vi "LeerBD.vi"(8 "error in (no error)":errorcluster) -> (0 "error out":errorcluster, 2 "BD":T1={"niv_presion_son_ref"=97.0, "Incertidumbre"="", "Tol +"="", "Tol -"="", "max_niv_ref"=97.0, "min_niv_ref"=97.0}, 3 "Prueba06 out":refnum<class "Prueba06.lvclass">)   [LabVIEW 2019, in "Prueba06.lvclass"]
uses:
  Prueba06.lvclass
  BD.ctl
  Base de Datos/SQLiteConnector/SQLiteConnection.lvclass
  Base de Datos/Base de Datos.lvclass
panel:
  in  "Tipo Equipo":enum16{"Sonometro", "Calibrador", "Dosimetro"}(ring)
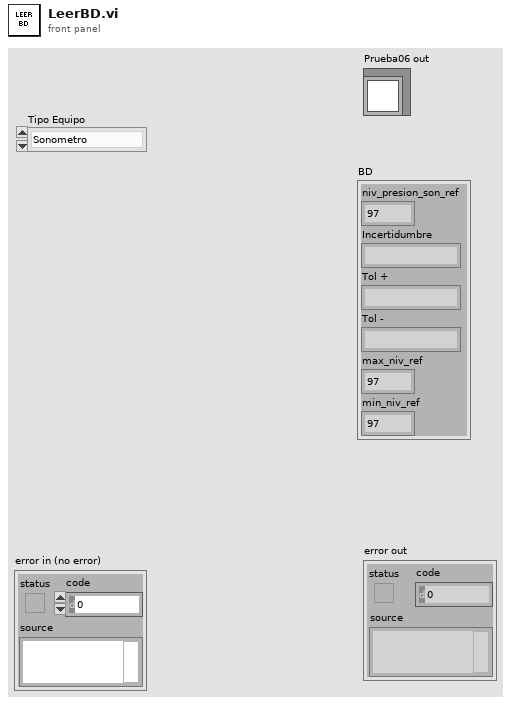
[diagram p1: front panel]
types:
  T1 = typedef "Prueba06.lvclass/BD.ctl" = cluster{"niv_presion_son_ref":dbl, "Incertidumbre":string, "Tol +":string, "Tol -":string, "max_niv_ref":dbl, "min_niv_ref":dbl}
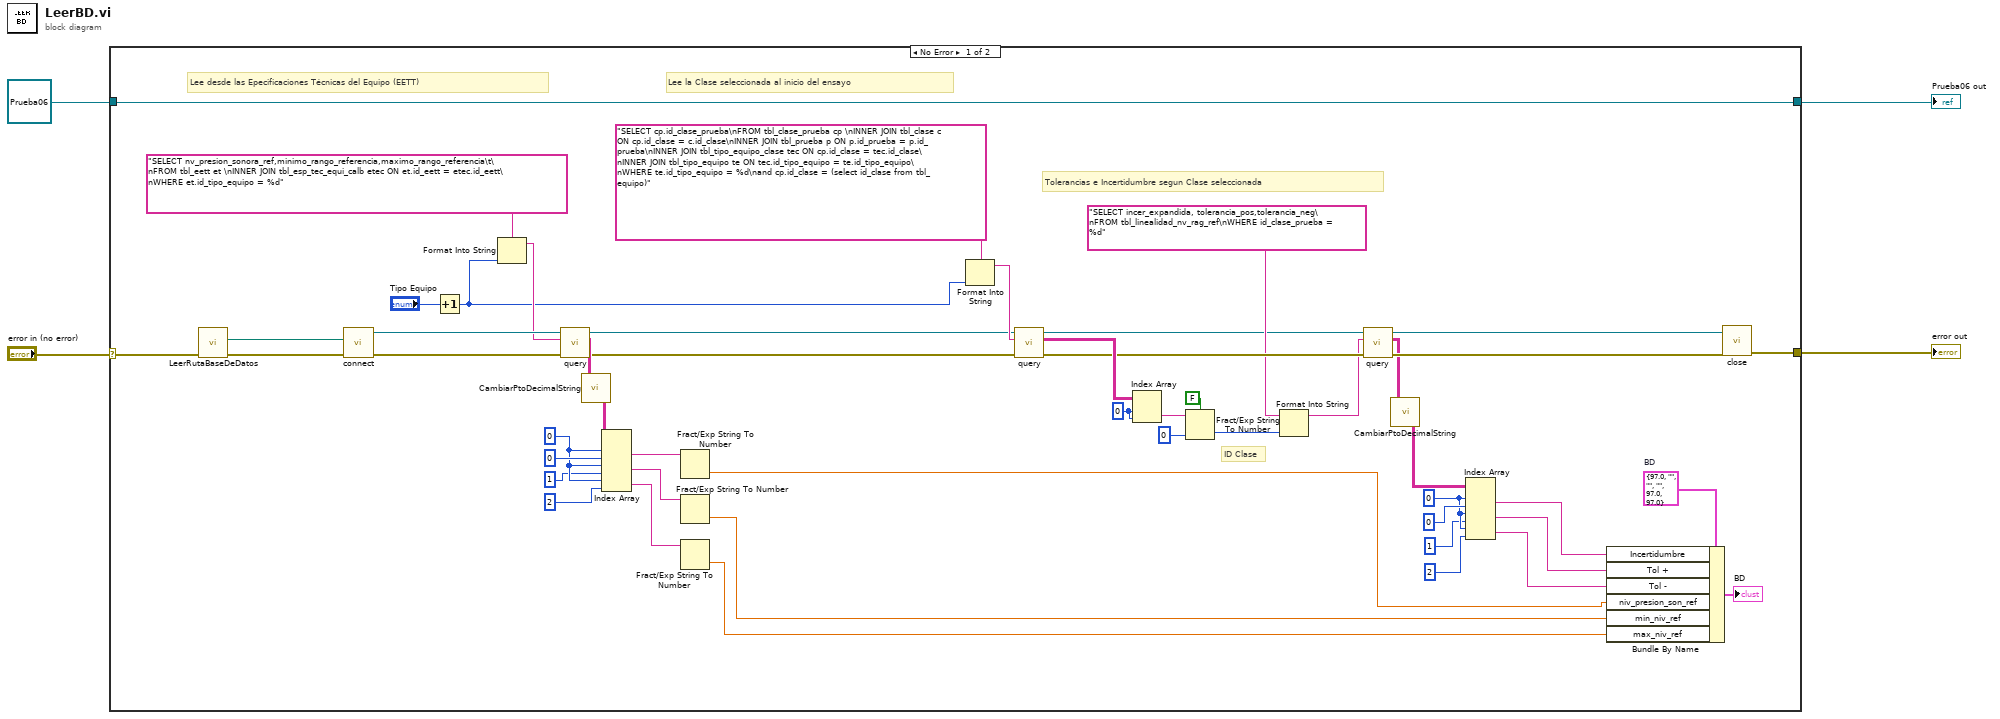
[diagram p0: block diagram]
diagram:
  n1 = case shown="No Error" "error in (no error)" {
    selector: "error in (no error)" -> [w46 w56]
    tunnel: [w32 w56] -> w3
    tunnel: [w54 w55] -> w1
    tunnel: refnum<class "Prueba06.lvclass"> refnum ("Prueba02 in") -> [w54 w55]
    frame No Error {
      w13 = 0 ("index (row)")
      w22 = T1 {"niv_presion_son_ref"=97.0, "Incertidumbre"="", "Tol +"="", "Tol -"="", "max_niv_ref"=97.0, "min_niv_ref"=97.0}  # BD
      w38 = 0 ("index (row)")
      w21 = 0 ("index (row)")
      # "Tolerancias e Incertidumbre segun Clase seleccionada"
      # "ID Clase"
      # "Lee la Clase seleccionada al inicio del ensayo"
      # "Lee desde las Epecificaciones Técnicas del Equipo (EETT)"
      n2 = call "LeerRutaBaseDeDatos.vi"("error in (no error)"=w46) -> ("error out"=w49:errorcluster, "Database Path"=w48:path)  [unwired: 9 in]
      n3 = call "connect.vi"("error in (no error)"=w49, "Database Path"=w48) -> ("error out"=w51:errorcluster, "object out"=w52:refnum<class "SQLiteConnection.lvclass">)  [unwired: 8 in]
      n4 = Increment(x="Tipo Equipo") -> (x+1=w27:enum16{"Sonometro", "Calibrador", "Dosimetro"})
      n5 = Format Into String(format string="SELECT nv_presion_sonora_ref,minimo_rango_referencia,maximo_rango_referencia\t\nFROM tbl_eett et \nINNER JOIN tbl_esp_tec_equi_calb etec ON et.id_eett = etec.id_eett\nWHERE et.id_tipo_equipo = %d", w27) -> (resulting string=w50:string)  [unwired: 2 in, 1 out]
      n6 = call "query.vi"("error in (no error)"=w51, "SQL Statement"=w50, "object in"=w52) -> ("error out"=w39:errorcluster, "result"=w43:string[][], "object out"=w40:refnum<class "SQLiteConnection.lvclass">)  [unwired: 5 in, 1 out]
      n7 = call "CambiarPtoDecimalString.vi"("result"=w43) -> ("result out"=w6:string[][])
      n8 = Index Array(array=w6, index (row) #1=w21, index (col) #1=0 ("disabled index (col)"), index (row) #2=w21, index (col) #2=1 ("disabled index (col)"), index (row) #3=w21, index (col) #3=2 ("disabled index (col)")) -> (element #1=w44:string, element #2=w18:string, element #3=w17:string)
      n9 = Fract/Exp String To Number(string=w44) -> (number=w23:dbl)  [unwired: 3 in, 1 out]
      n10 = Fract/Exp String To Number(string=w18) -> (number=w16:dbl)  [unwired: 3 in, 1 out]
      n11 = Fract/Exp String To Number(string=w17) -> (number=w15:dbl)  [unwired: 3 in, 1 out]
      n12 = Format Into String(format string="SELECT cp.id_clase_prueba\nFROM tbl_clase_prueba cp \nINNER JOIN tbl_clase c ON cp.id_clase = c.id_clase\nINNER JOIN tbl_prueba p ON p.id_prueba = p.id_prueba\nINNER JOIN tbl_tipo_equipo_clase tec ON cp.id_clase = tec.id_clase\nINNER JOIN tbl_tipo_equipo te ON tec.id_tipo_equipo = te.id_tipo_equipo\nWHERE te.id_tipo_equipo = %d\nand cp.id_clase = (select id_clase from tbl_equipo)", w27) -> (resulting string=w41:string)  [unwired: 2 in, 1 out]
      n13 = call "query.vi"("error in (no error)"=w39, "SQL Statement"=w41, "object in"=w40) -> ("error out"=w33:errorcluster, "result"=w34:string[][], "object out"=w29:refnum<class "SQLiteConnection.lvclass">)  [unwired: 5 in, 1 out]
      n14 = Index Array(array=w34, index (row)=w38, index (col)=w38) -> (element=w36:string)
      n15 = Fract/Exp String To Number(use system decimal point (T)=FALSE, string=w36, default (0 dbl)=0 ("index (row)")) -> (number=w24:i32)  [unwired: 1 in, 1 out]
      n16 = Format Into String(format string="SELECT incer_expandida, tolerancia_pos,tolerancia_neg\nFROM tbl_linealidad_nv_rag_ref\nWHERE id_clase_prueba = %d", w24) -> (resulting string=w28:string)  [unwired: 2 in, 1 out]
      n17 = call "query.vi"("error in (no error)"=w33, "SQL Statement"=w28, "object in"=w29) -> ("error out"=w30:errorcluster, "result"=w26:string[][], "object out"=w25:refnum<class "SQLiteConnection.lvclass">)  [unwired: 5 in, 1 out]
      n18 = call "CambiarPtoDecimalString.vi"("result"=w26) -> ("result out"=w5:string[][])
      n19 = Index Array(array=w5, index (row) #1=w13, index (col) #1=0 ("disabled index (col)"), index (row) #2=w13, index (col) #2=1 ("disabled index (col)"), index (row) #3=w13, index (col) #3=2 ("disabled index (col)")) -> (element #1=w10:string, element #2=w9:string, element #3=w8:string)
      n20 = Bundle By Name(cluster=w22, "Incertidumbre"=w10, "Tol +"=w9, "Tol -"=w8, "niv_presion_son_ref"=w23, "min_niv_ref"=w16, "max_niv_ref"=w15) -> (→"BD":T1)
      n21 = call-dynamic "close.vi"("error in (no error)"=w30, "object in"=w25) -> ("error out"=w32:errorcluster)  [unwired: 8 in, 1 out]
    }
    frame Error {
    }
  }
  "error out" <- w3
  "Prueba06 out" <- w1
